vi "GetInstVisaHandle.vi"(8 "error in (no error)":errorcluster, 11 "NetA_RSZVL in":refnum<class "NetA_RSZVL.lvclass">) -> (0 "error out":errorcluster, 2 "VISA resource name out":refnum<visa-resource-name>, 3 "NetA_RSZVL out":refnum<class "NetA_RSZVL.lvclass">)   [LabVIEW 2014, in "NetA_RSZVL.lvclass"]
uses:
  NetA_RSZVL.lvclass
  NetA_RSZVL.lvclass/NetA_RSZVL.ctl
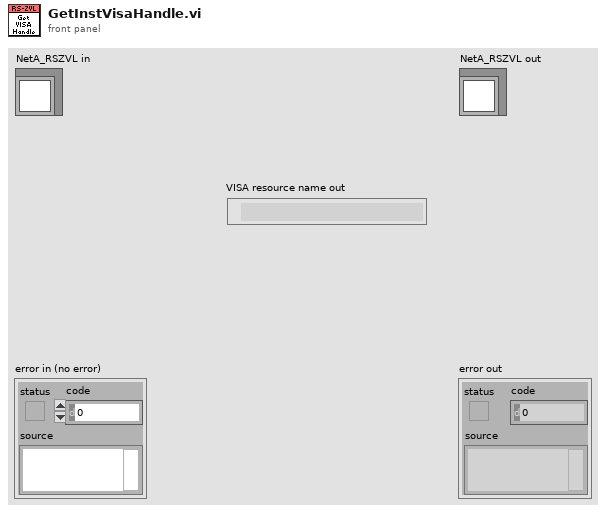
[diagram p1: front panel]
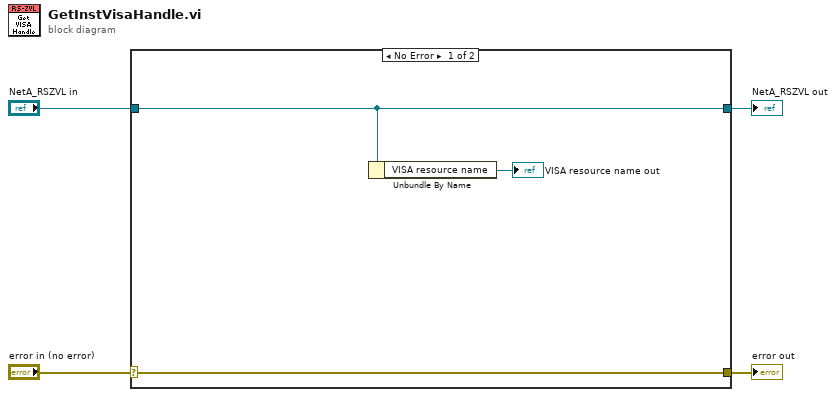
[diagram p0: block diagram]
diagram:
  n1 = case shown="No Error" "error in (no error)" {
    selector: "error in (no error)" -> [w7 w9]
    tunnel: [w7 w9] -> w3
    tunnel: [w6 w8] -> w1
    tunnel: "NetA_RSZVL in" -> [w6 w8]
    frame No Error {
      n2 = Unbundle By Name(w6) -> ("VISA resource name"=→"VISA resource name out":refnum<visa-resource-name>)
    }
    frame Error {
    }
  }
  "error out" <- w3
  "NetA_RSZVL out" <- w1
